vi "Write Global Locked.vi"(8 "error in (no error)":errorcluster, 10 "Global":refnum<class "System.lvclass">, 11 "DriveMotorsLeft in":refnum<class "DriveMotorsLeft.lvclass">) -> (0 "error out":errorcluster, 3 "DriveMotorsLeft out":refnum<class "DriveMotorsLeft.lvclass">)   [LabVIEW 2013]
uses:
  Robot Global Data.vi
  DriveMotorsLeft.lvclass
  System/System.lvclass
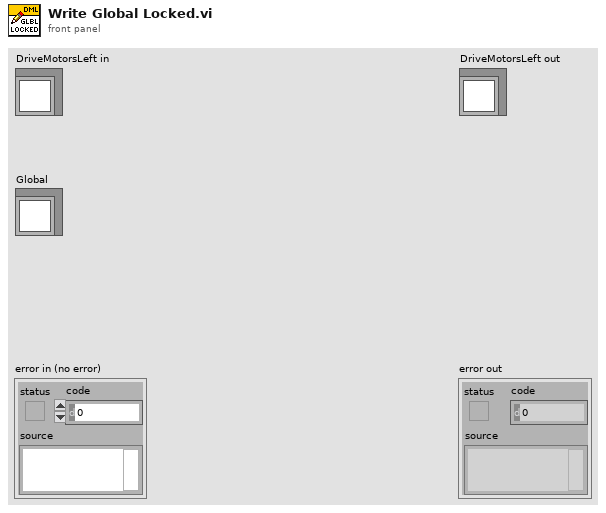
[diagram p1: front panel]
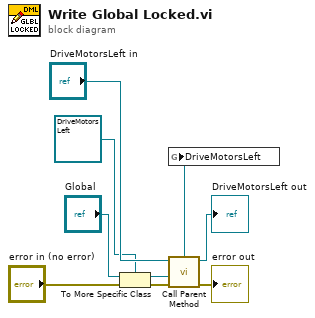
[diagram p0: block diagram]
diagram:
  n1 = To More Specific Class(target class=refnum<class "DriveMotorsLeft.lvclass"> refnum ("DriveMotorsLeft.lvclass"), reference="Global", error in="error in (no error)") -> (specific class reference=w3:refnum<class "DriveMotorsLeft.lvclass">, error out=w1:errorcluster)
  n2 = global write "Robot Global Data.vi" "DriveMotorsLeft"(w3) -> ()
  n3 = call-parent "Call Parent Method"("error in (no error)"=w1, "System in"="DriveMotorsLeft in") -> ("error out"=→"error out":errorcluster, "System out"=→"DriveMotorsLeft out":refnum<class "DriveMotorsLeft.lvclass">)  [unwired: 8 in]
